vi "Get Upper BandLimit.vi"(8 "error in (no error)":errorcluster, 11 "VISA resource name":refnum<visa-resource-name>) -> (0 "error out":errorcluster, 1 "UpperBand (out)":dbl, 3 "VISA resource name out":refnum<visa-resource-name>)   [LabVIEW 2018, in "JULABO DeviceDriver.lvlib"]
doc: "This VI returns the adjusted maximum allowed difference between internal and external temperature during heating up.\n\nNote:\nThis function is not available for instruments which does not support different values for upper and lower bandlimit. Please use <B>JULABO_Data_GetBand.vi</B> in case your instrument supports only one bandlimit. See operating manual to check whether your instrument supperts different values for lower and upper bandlimit.\n\nThis function is not available for devices which does not have an external sensor plug."
uses:
  JULABO DeviceDriver.lvlib
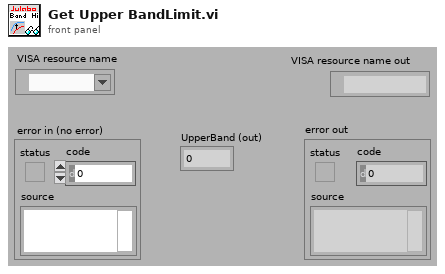
[diagram p1: front panel]
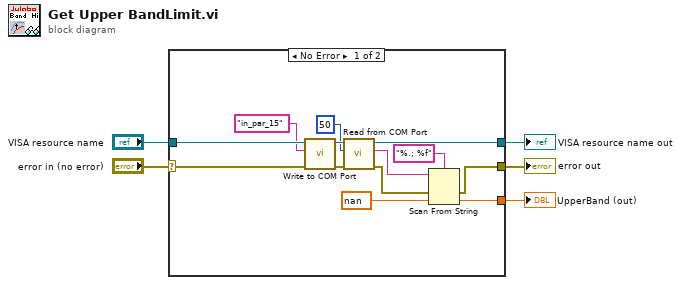
[diagram p0: block diagram]
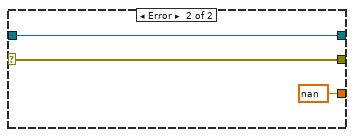
[diagram p2: hidden frame]
diagram:
  n1 = case shown="No Error" "error in (no error)" {
    selector: "error in (no error)" -> [w17 w20]
    tunnel: "VISA resource name" -> [w18 w21]
    tunnel: [w16 w20] -> w3
    tunnel: [w15 w21] -> w2
    tunnel: [w7 nan] -> w1
    frame No Error {
      n2 = call "Write to COM Port.vi"("error in"=w17, "Command (input)"="in_par_15", "VISA resource name in"=w18) -> ("error out"=w14:errorcluster, "VISA resource name out"=w13:refnum<visa-resource-name>)  [unwired: 7 in]
      n3 = call "Read from COM Port.vi"("error in"=w14, "Byte to Read (-1:All)"=u32 50 ("Anzahl der Byte"), "VISA resource name in"=w13) -> ("error out"=w11:errorcluster, "String (output)"=w10:string, "VISA resource name out"=w15:refnum<visa-resource-name>)  [unwired: 5 in, 1 out]
      n4 = Scan From String(format string="%.; %f" ("Format-String"), input string=w10, error in=w11, default 1=nan ("Standardwert1")) -> (error out=w16:errorcluster, output 1=w7:dbl)  [unwired: 1 in, 2 out]
    }
    frame Error {
    }
  }
  "error out" <- w3
  "VISA resource name out" <- w2
  "UpperBand (out)" <- w1
